vi "Error 5005.vi"(8 "error in (no error)":errorcluster) -> (0 "error out":errorcluster)   [LabVIEW 2019, in "gRPC Template Creation Utility.lvlib"]
uses:
  gRPC Template Creation Utility.lvlib
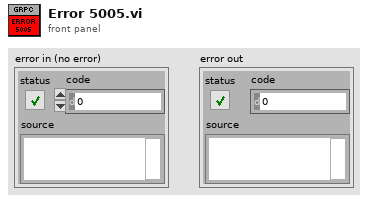
[diagram p1: front panel]
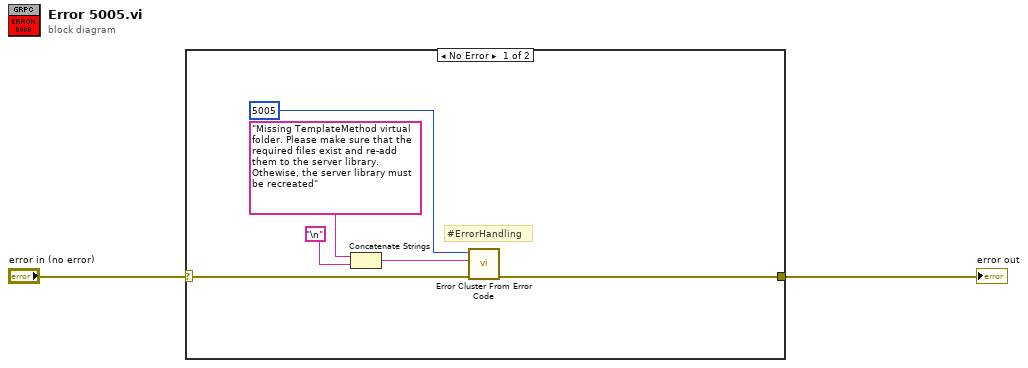
[diagram p0: block diagram]
diagram:
  n1 = case shown="No Error" "error in (no error)" {
    selector: "error in (no error)" -> [w3 w9]
    tunnel: [w8 w9] -> w2
    frame No Error {
      # "#ErrorHandling"
      n2 = Concatenate Strings("Missing TemplateMethod virtual folder. Please make sure that the required files exist and re-add them to the server library. Othewise, the server library must be recreated" ("error message (\"\")"), "\n") -> (w7:string)
      n3 = call <vilib>:"Error Cluster From Error Code.vi"("error in (no error)"=w3, "error message (\"\")"=w7, "error code (0)"=5005) -> ("error out"=w8:errorcluster)  [unwired: 6 in]
    }
    frame Error {
    }
  }
  "error out" <- w2
